vi "Create Symbol Loader Factory.vi"(8 "error in (no error)":errorcluster, 11 "TwinCAT ADS in":refnum<class "TwinCAT ADS.lvclass">) -> (0 "error out":errorcluster, 3 "TwinCAT ADS out":refnum<class "TwinCAT ADS.lvclass">)   [LabVIEW 2018, in "TwinCAT ADS.lvclass"]
uses:
  TwinCAT ADS.lvclass
  TwinCAT.Ads
  TwinCAT ADS.lvclass/TwinCAT ADS.ctl
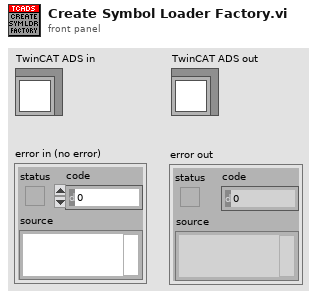
[diagram p1: front panel]
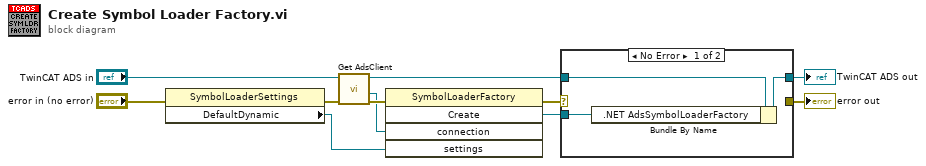
[diagram p0: block diagram]
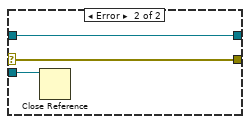
[diagram p2: hidden frame]
diagram:
  n1 = property class="SymbolLoaderSettings"(error in="error in (no error)") -> (error out=w10:errorcluster, "DefaultDynamic"=w1:refnum<k24>)  [unwired: 1 in, 1 out]
  n2 = call "Get AdsClient.vi"("error in (no error)"=w10, "TwinCAT ADS in"="TwinCAT ADS in") -> ("error out"=w11:errorcluster, ".NET TcAdsClient refnum"=w7:refnum<k24>, "TwinCAT ADS out"=w6:refnum<class "TwinCAT ADS.lvclass">)  [unwired: 7 in]
  n3 = invoke class="SymbolLoaderFactory" method="Create"(error in=w11, "connection"=w7, "settings"=w1) -> (error out=w3:errorcluster, "Create"=w5:refnum<k24>)  [unwired: 2 in, 3 out]
  n4 = case shown="No Error" w3 {
    selector: w3 -> [_ w16]
    tunnel: w6 -> [w14 w17]
    tunnel: w5 -> [w13 w15]
    tunnel: [w12 w17] -> w4
    tunnel: [_ w16] -> w2
    frame No Error {
      n5 = Bundle By Name(cluster=w14, ".NET AdsSymbolLoaderFactory"=w13) -> (w12:refnum<class "TwinCAT ADS.lvclass">)
    }
    frame Error {
      n6 = Close Reference(reference=w15) -> ()  [unwired: 1 in, 1 out]
    }
  }
  "error out" <- w2
  "TwinCAT ADS out" <- w4
